vi "Write ColorGridCoords.vi"(8 "error in (no error)":errorcluster, 10 "ColorGridCoords":T1, 11 "ColorSelector in":refnum<class "ColorSelector.lvclass">) -> (0 "error out":errorcluster, 3 "ColorSelector out":refnum<class "ColorSelector.lvclass">)   [LabVIEW 2015, in "ColorSelector.lvclass"]
doc: "Writes the current ColorGridCoords to the State Data.\n<b> </b> <b> </b>\n©2017 Q Software Innovations, LLC (QSI)\nwritten by Quentin Alldredge\nproduced in LabVIEW 2015\n\nsupport@qsoftwareinnovations.com\nwww.qsoftwareinnovations.com\n\nAll rights reserved.\n\nRedistribution and use in source and binary forms, with or without modification, are permitted provided that the following conditions are met:\n\n * Redistributions of source code must retain the above copyright notice, this list of conditions and the following disclaimer.\n * Redistributions in binary form must reproduce the above copyright notice, this list of conditions and the following disclaimer in the documentation and/or other materials provided with the distribution.\n * Neither the name of Q Software Innovations, LLC. nor the names of its contributors may be used to endorse or promote products derived from this software without specific prior written permission.\n\nTHIS SOFTWARE IS PROVIDED BY THE COPYRIGHT HOLDERS AND CONTRIBUTORS \"AS IS\" AND ANY EXPRESS OR IMPLIED WARRANTIES, INCLUDING, BUT NOT LIMITED TO, THE IMPLIED WARRANTIES OF MERCHANTABILITY AND FITNESS FOR A PARTICULAR PURPOSE ARE DISCLAIMED. IN NO EVENT SHALL THE COPYRIGHT OWNER OR CONTRIBUTORS BE LIABLE FOR ANY DIRECT, INDIRECT, INCIDENTAL, SPECIAL, EXEMPLARY, OR CONSEQUENTIAL DAMAGES (INCLUDING, BUT NOT LIMITED TO, PROCUREMENT OF SUBSTITUTE GOODS OR SERVICES; LOSS OF USE, DATA, OR PROFITS; OR BUSINESS INTERRUPTION) HOWEVER CAUSED AND ON ANY THEORY OF LIABILITY, WHETHER IN CONTRACT, STRICT LIABILITY, OR TORT (INCLUDING NEGLIGENCE OR OTHERWISE) ARISING IN ANY WAY OUT OF THE USE OF THIS SOFTWARE, EVEN IF ADVISED OF THE POSSIBILITY OF SUCH DAMAGE."
uses:
  ColorSelector.lvclass
  <vilib>/Utility/miscctls.llb/LVPoint32TypeDef.ctl
  ColorSelector.lvclass/ColorSelector.ctl
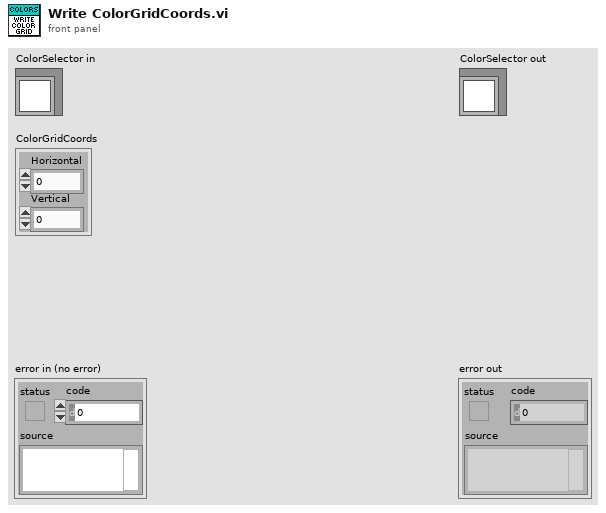
[diagram p1: front panel]
types:
  T1 = typedef "LVPoint32TypeDef.ctl" = cluster{"Horizontal":i32, "Vertical":i32}
  T2 = typedef "ColorSelector.lvclass/State Data.ctl" = cluster{"Hue[]":u32[], "GreySelectPic":picture, "ColorSelectPic":picture, "ActiveSelector":T3, "ColorGridCoords":T1, "GreyGridCoords":T1}
  T3 = typedef "ColorSelector.lvclass/Active Selector Enum.ctl" = enum16{"Grey", "Color"}
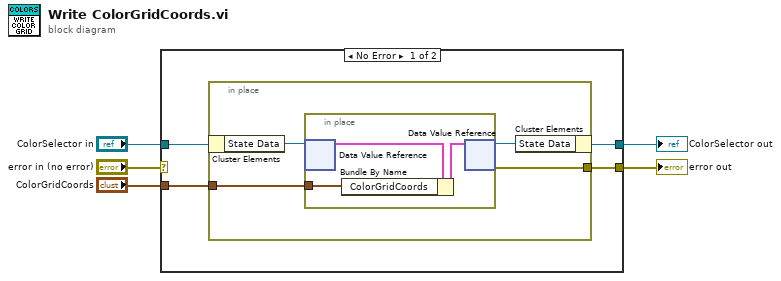
[diagram p0: block diagram]
diagram:
  n1 = case shown="No Error" "error in (no error)" {
    selector: "error in (no error)" -> [_ w18]
    tunnel: [w7 w18] -> w4
    tunnel: [w8 w17] -> w2
    tunnel: "ColorSelector in" -> [w9 w17]
    tunnel: "ColorGridCoords" -> [w6 _]
    frame No Error {
      n2 = in-place {
        in-place-border: [w11] -> w7
        in-place-border: w6 -> [w10]
        n3 = in-place-cluster #1(w9) -> ("State Data"=w13:refnum<data-value>)
        n4 = in-place {
          in-place-border: w10 -> [w16]
          n5 = in-place-dvr #2(w13) -> (w15:T2)  [unwired: 1 out]
          n6 = Bundle By Name(cluster=w15, "ColorGridCoords"=w16) -> (w14:T2)
          n7 = in-place-dvr #2(w14) -> (w12:refnum<data-value>, w11:errorcluster)
        }
        n8 = in-place-cluster #1("State Data"=w12) -> (w8:refnum<class "ColorSelector.lvclass">)
      }
    }
    frame Error {
    }
  }
  "error out" <- w4
  "ColorSelector out" <- w2
